vi "avreager based on sub vi.vi"() -> ()   [LabVIEW 2020]
panel:
  out "(a+b)/2":dbl
  in  "b":dbl
  in  "a":dbl
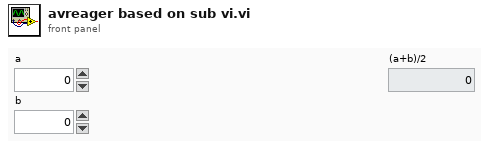
[diagram p1: front panel]
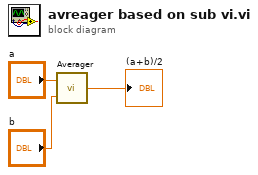
[diagram p0: block diagram]
diagram:
  n1 = call "Averager.vi"("b"="b", "a"="a") -> ("(a+b)/2"=→"(a+b)/2":dbl)
